vi "Extract Most Significant Orders.vi"(6 "window info":T1={"window type"=10, "window length"=2048} {"window type" items=["None"=0, "Hanning"=1, "Hamming"=2, "Blackman-Harris"=3, "Exact Blackman"=4, "Blackman"=5, "Flat Top"=6, "4 Term B-Harris"=7, "7 Term B-Harris"=8, "Low Sidelobe"=9, "Gaussian"=62]; "window length" min=0}, 7 "bandwidth":T2={"bandwidth value"=0.5, "bandwidth unit"=enum."Order"} {"bandwidth value" min=0.0 format="%.2f"}, 8 "error in (no error)":errorcluster, 9 "number of orders (3)":i32=3, 10 "speed profile":T3 {"speed [RPM]" format="%.2f"; "time [s]" format="%.2f"}, 11 "scaled signal [EU]":waveform(dbl)={"t0"=timestamp(0 s since 1904-01-01), "dt"=0.0, "Y"=[]}) -> (0 "error out":errorcluster, 1 "unit label":string, 2 "orders":dbl[](array[numeric]) format="%.2f", 3 "order waveforms [EU]":waveform(dbl)[](array[waveform]), 4 "actual window":T1={"window type"=10, "window length"=2048} {"window type" items=["None"=0, "Hanning"=1, "Hamming"=2, "Blackman-Harris"=3, "Exact Blackman"=4, "Blackman"=5, "Flat Top"=6, "4 Term B-Harris"=7, "7 Term B-Harris"=8, "Low Sidelobe"=9, "Gaussian"=62]; "window length" min=0})   [LabVIEW 2017]
doc: "Extracts the orders with the highest power."
uses:
  <vilib>/addons/Sound and Vibration/Order Analysis/Tach Process/SubVIs/speed profile.ctl
  <vilib>/addons/Sound and Vibration/Order Analysis/Ref Gabor Order Tracking/Mask Bandwidth.ctl
  <vilib>/addons/Sound and Vibration/Order Analysis/Ref Gabor Order Tracking/window information.ctl
  <vilib>/addons/Sound and Vibration/Order Analysis/Ref Gabor Order Tracking/Get Order-RPM Spectral Map (DBL).vi
  <vilib>/addons/_NISVFA/_Shared subVIs/Common/svc_Engineering Units to Unit Label.vi
  <vilib>/addons/_NISVFA/_Shared subVIs/Common/svc_Unit Label to Engineering Units.vi
  <vilib>/addons/Sound and Vibration/Order Analysis/Gabor Order Tracking/SoundVib_Gabor.lvlib
  <vilib>/addons/Sound and Vibration/Order Analysis/Tach Process/SoundVib_TachProcess.lvlib
panel:
  # "Extract Most Significant Orders"
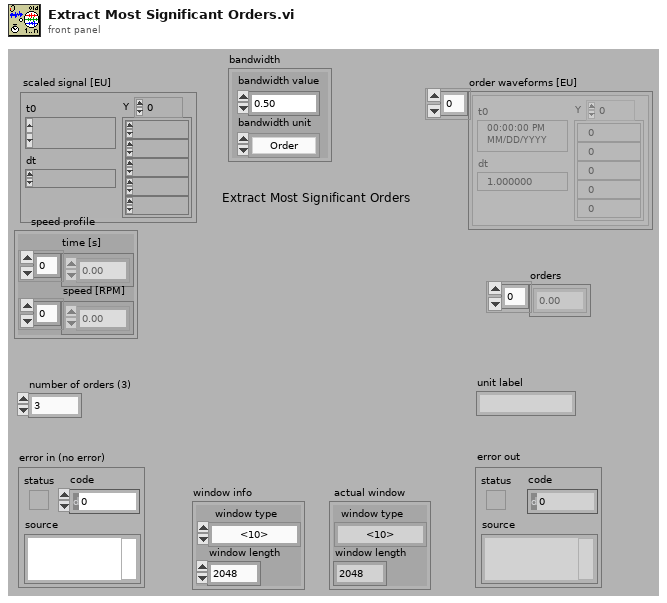
[diagram p1: front panel]
types:
  T1 = typedef "SoundVib_Gabor.lvlib/window information.ctl" = cluster{"window type":u32, "window length":i32}
  T2 = typedef "SoundVib_Gabor.lvlib/Mask Bandwidth.ctl" = cluster{"bandwidth value":dbl, "bandwidth unit":enum16{"Order", "Hz"}}
  T3 = typedef "SoundVib_TachProcess.lvlib/speed profile.ctl" = cluster{"time [s]":dbl[], "speed [RPM]":dbl[]}
  T4 = cluster{"minimum":dbl, "maximum":dbl, "increment":dbl}
  T5 = typedef "svc_Channel Info.ctl" = cluster{"sensor sensitivity":dbl, "engineering units":T6, "dB reference":dbl, "custom label":string, "weighting filter":T7, "pregain":dbl}
  T6 = typedef "svc_Engineering Units Text Ring.ctl" = u16
  T7 = typedef "svc_Weighting Filter Text Ring.ctl" = u16
  T8 = typedef "SoundVib_Gabor.lvlib/GT RefNum.ctl" = refnum<k1>
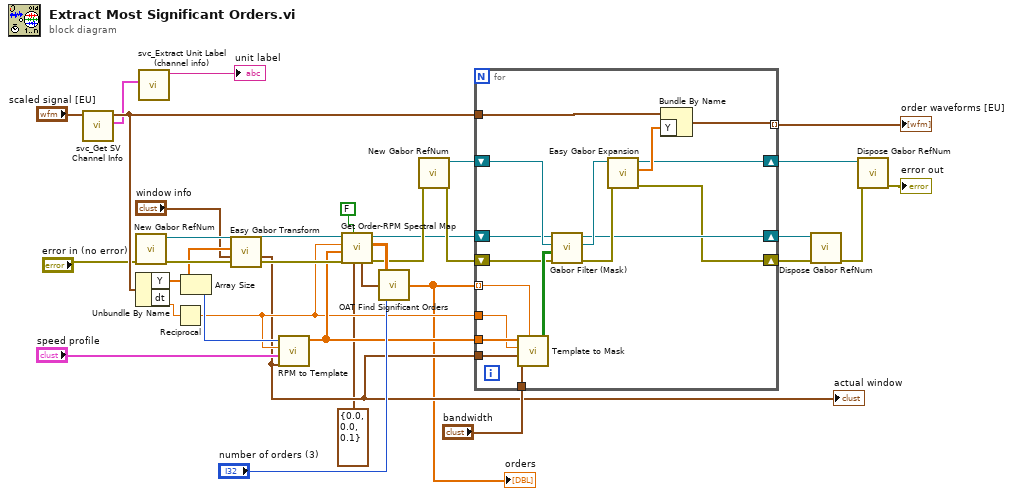
[diagram p0: block diagram]
diagram:
  n1 = call <vilib>:"svc_Get SV Channel Info.vi"("scaled signal [EU]"="scaled signal [EU]") -> ("channel info"=w8:T5, "dup scaled signal [EU]"=w9:waveform(dbl))  [unwired: 5 in, 4 out]
  n2 = call <vilib>:"New Gabor RefNum.vi"("error in (no error)"="error in (no error)") -> ("error out"=w33:errorcluster, "RefNum"=w34:T8)  [unwired: 8 in]
  n3 = Unbundle By Name(w9) -> ("Y"=w16:dbl[], "dt"=w15:dbl)
  n4 = call <vilib>:"svc_Extract Unit Label (channel info).vi"("channel info"=w8) -> ("unit label"=→"unit label":string)  [unwired: 8 in, 2 out]
  n5 = Reciprocal(x=w15) -> (1/x=w14:dbl)
  n6 = Array Size(array=w16) -> (size(s)=w24:i32)
  n7 = call <vilib>:"Easy Gabor Transform.vi"("error in (no error)"=w33, "window info"="window info", "x[n]"=w16, "RefNum in"=w34) -> ("error out"=w31:errorcluster, "actual window"=w11:T1, "RefNum out"=w32:T8)  [unwired: 3 in, 2 out]
  "actual window" <- w11
  n8 = call <vilib>:"RPM to Template.vi"("window info"=w11, "speed profile"="speed profile", "sampling frequency [Hz]"=w14, "signal length"=w24) -> ("Gabor template"=w19:dbl[])  [unwired: 6 in, 1 out]
  n9 = call-poly <vilib>:"Get Order-RPM Spectral Map.vi"("order range (auto)"=T4 {"minimum"=0.0, "maximum"=0.0, "increment"=0.1}, "dB On (T)"=FALSE ("log scale?"), "error in (no error)"=w31, "Gabor template"=w19, "sampling frequency [Hz]"=w14, "RefNum in"=w32) -> ("error out"=w26:errorcluster, "spectral map"=w29:dbl[][], "RefNum out"=w2:T8, "order scale"=w28:cluster{"offset":dbl, "multiplier":dbl})  [unwired: 2 out]
  n10 = call <vilib>:"OAT Find Significant Orders.vi"("num of significant orders"="number of orders (3)", "order scale"=w28, "order spectrum"=w29) -> ("orders"=w6:dbl[])
  "orders" <- w6
  n11 = call <vilib>:"New Gabor RefNum.vi"("error in (no error)"=w26) -> ("error out"=w25:errorcluster, "RefNum"=w4:T8)  [unwired: 8 in]
  n12 = for {
    tunnel: w19 -> [w51]
    shift-right: [w35] -> w22
    shift-left: w25 -> [w48]
    tunnel: w6 -> [w49] mode=indexing
    tunnel: w11 -> [w45]
    tunnel: "bandwidth" -> [w44]
    tunnel: w14 -> [w43]
    tunnel: w9 -> [w41]
    tunnel: [w40] -> w17 mode=indexing
    shift-right: [w36] -> w3
    shift-left: w4 -> [w39]
    shift-right: [w37] -> w1
    shift-left: w2 -> [w38]
    n13 = call <vilib>:"Template to Mask.vi"("order (1.0)"=w49, "bandwidth"=w44, "window info"=w45, "sampling frequency [S/s]"=w43, "Gabor template"=w51) -> ("mask array"=w50:bool[][])  [unwired: 6 in]
    n14 = call <vilib>:"Gabor Filter (Mask).vi"("error in (no error)"=w48, "mask array"=w50, "dest RefNum in"=w39, "src RefNum in"=w38) -> ("error out"=w46:errorcluster, "dest RefNum out"=w47:T8, "RefNum out"=w37:T8)  [unwired: 5 in]
    n15 = call <vilib>:"Easy Gabor Expansion.vi"("error in (no error)"=w46, "RefNum in"=w47) -> ("error out"=w35:errorcluster, "time waveform"=w42:dbl[], "RefNum out"=w36:T8)  [unwired: 7 in]
    n16 = Bundle By Name(cluster=w41, "Y"=w42) -> (w40:waveform(dbl))
  }
  "order waveforms [EU]" <- w17
  n17 = call <vilib>:"Dispose Gabor RefNum.vi"("error in (no error)"=w22, "RefNum in"=w1) -> ("error out"=w23:errorcluster)  [unwired: 6 in]
  n18 = call <vilib>:"Dispose Gabor RefNum.vi"("error in (no error)"=w23, "RefNum in"=w3) -> ("error out"=→"error out":errorcluster)  [unwired: 6 in]
